vi "After Launch Init Core.vi"(8 "error in (no error)":errorcluster, 11 "CS++GoBangServer in":refnum<class "CS++GoBangServer.lvclass">) -> (0 "error out":errorcluster, 3 "CS++GoBangServer out":refnum<class "CS++GoBangServer.lvclass">)   [LabVIEW 2014, in "GoBang.lvlib" / "CS++GoBangServer.lvclass"]
doc: "Use <b>Pre Launch init.vi</b> method only for sanity checks that are supposed to prevent the actor from launching if they fail. Use <B>this</B> method instead to initialize unique resources that must be released during the <b>Stop Core.vi</b> method. A corresponding high priority message will become dispatched before the <B>Actor Framework.lvlib:Actor.lvclass.Actor Core.vi</b> is called.\n\n<b>Derived classed should call the parent methode first</b> and their own initialization code after.\n\nRefer also to the ongoing discussion at https://decibel.ni.com/content/message/57394#57394."
uses:
  CS++GoBangServer.lvclass
  CS++GoBangServer.lvclass/CS++GoBangServer.ctl
  CSPP_Core/Classes/CS++ProcessVariables/PVConnection/PVConnection.lvclass/PVConnection.ctl
  CSPP_Core/Classes/CS++ProcessVariables/ProcessVariable/PV.lvclass/PV.ctl
  CSPP_Core/Actors/CS++BaseActor/CS++BaseActor.lvclass
  CSPP_Core/Classes/CS++ProcessVariables/ProcessVariable/PV.lvclass
  GoBang.lvlib
  CSPP_Core/Classes/CS++ProcessVariables/PVConnection/PVConnection.lvclass
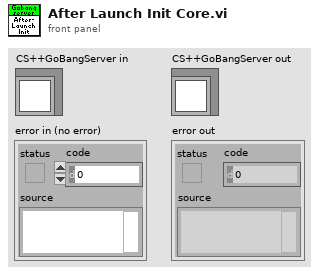
[diagram p1: front panel]
types:
  T1 = cluster{"Write Access":enum8{"Allowed", "Required", "None"}, "Read Access":enum8{"Allowed", "Required", "None"}}
  T2 = cluster{"BlackPlayer":refnum<class "PVConnection.lvclass">, "WhitePlayer":refnum<class "PVConnection.lvclass">, "GameBoard":refnum<class "PVConnection.lvclass">, "GameState":refnum<class "PVConnection.lvclass">}
  T3 = cluster{"[0]":refnum<class "PVConnection.lvclass">, "[1]":refnum<class "PVConnection.lvclass">, "[2]":refnum<class "PVConnection.lvclass">, "[3]":refnum<class "PVConnection.lvclass">}
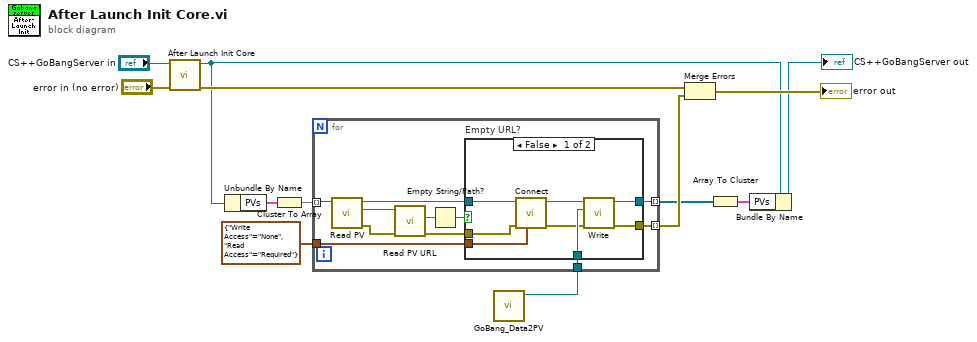
[diagram p0: block diagram]
diagram:
  n1 = call-parent "After Launch Init Core.vi"("error in (no error)"="error in (no error)", "CS++BaseActor in"="CS++GoBangServer in") -> ("error out"=w6:errorcluster, "CS++BaseActor out"=w3:refnum<class "CS++GoBangServer.lvclass">)  [unwired: 8 in]
  n2 = Unbundle By Name(w3) -> ("PVs"=w7:T2)
  n3 = Cluster To Array(cluster=w7) -> (array=w9:refnum<class "PVConnection.lvclass">[])
  n4 = call "GoBang_Data2PV.vi"() -> ("PV out"=w1:refnum<class "PV.lvclass">)  [unwired: 11 in]
  n5 = for {
    tunnel: w9 -> [w19] mode=indexing
    tunnel: T1 {"Write Access"=enum."None", "Read Access"=enum."Required"} ("Access") -> [w24]
    tunnel: [w23] -> w10 mode=indexing
    tunnel: [w21] -> w11 mode=indexing
    tunnel: w1 -> [w20]
    n6 = call "Read PV.vi"("PVConnection in"=w19) -> ("error out"=w17:errorcluster, "PV"=w18:refnum<class "PV.lvclass">, "PVConnection out"=w14:refnum<class "PVConnection.lvclass">)  [unwired: 8 in]
    n7 = call "Read PV URL.vi"("error in (no error)"=w17, "PV in"=w18) -> ("error out"=w15:errorcluster, "PV URL"=w16:string)  [unwired: 7 in, 1 out]
    n8 = Empty String/Path?(string/path=w16) -> (empty?=w22:bool)
    n9 = case "Empty URL?" shown="False" w22 {
      tunnel: w14 -> [w32 w33]
      tunnel: w24 -> [w31 _]
      tunnel: [w26 w33] -> w23
      tunnel: [w25 _] -> w21
      tunnel: w15 -> [w30 _]
      tunnel: w20 -> [w29 _]
      frame False {
        n10 = call "Connect.vi"("Access (R/W allowed)"=w31, "error in (no error)"=w30, "PVConnection in"=w32) -> ("error out"=w28:errorcluster, "PVConnection out"=w27:refnum<class "PVConnection.lvclass">)  [unwired: 7 in]
        n11 = call "Write.vi"("error in (no error)"=w28, "PV"=w29, "PVConnection in"=w27) -> ("error out"=w25:errorcluster, "PVConnection out"=w26:refnum<class "PVConnection.lvclass">)  [unwired: 7 in]
      }
      frame True {
      }
    }
  }
  n12 = Merge Errors(w6, w11) -> (→"error out":errorcluster)
  n13 = Array To Cluster(array=w10) -> (cluster=w8:T3)
  n14 = Bundle By Name(cluster=w3, "PVs"=w8) -> (→"CS++GoBangServer out":refnum<class "CS++GoBangServer.lvclass">)
